vi "Constants.vi"   [LabVIEW 2023, in "UDPlog.lvlib" / "UDPlog Transceiver.lvclass"]
uses:
  UDPlog Transceiver.lvclass
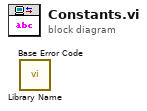
[diagram p0: block diagram]
diagram:
  n1 = call "Library Name.vi"() -> ()  [unwired: 11 in, 1 out]
  n2 = call "Base Error Code.vi"() -> ()  [unwired: 11 in, 1 out]
